vi "Connect.vi"(5 "Connect Meta":T4={"QoS"=enum."At most once", "DUP"=FALSE, "Retain"=TRUE, "Keep Alive (sec)"=60}, 6 "Client ID":string="LabVIEW_MQTT_Client", 7 "Connect Flags":T7, 8 "error in (no error)":errorcluster, 9 "Will Info":T5={"Will Topic"="Will Topic", "Will Message"="Last Will"}, 10 "User Info":T6={"Username"="User", "Password"="password"}, 11 "MQTT Broker":cluster{"address (IP)":string, "port":u16}={"address (IP)"="broker.mqttdashboard.com", "port"=1883}) -> (0 "error out":errorcluster, 2 "Connection Status":T1=enum."Connection refused: not authorized", 3 "connection ID out":refnum<k5>)   [LabVIEW 2025, in "DAQIO MQTT.lvlib"]
doc: "Connects to an MQTT broker server with required settings. \n\n© 2015 - daq.io, LLC - Peter Adelhardt"
uses:
  DAQIO MQTT.lvlib
  Controls/Connect Flags.ctl
  Controls/User Info.ctl
  Controls/Will Info.ctl
  Controls/DUP_Flag.ctl
  Controls/Retain_Flag.ctl
  Controls/Connection_Return_Codes.ctl
  Controls/Conn_FGV_Cmds.ctl
  Controls/Conn_Stat_FGV_Cmds.ctl
  Controls/MessageType.ctl
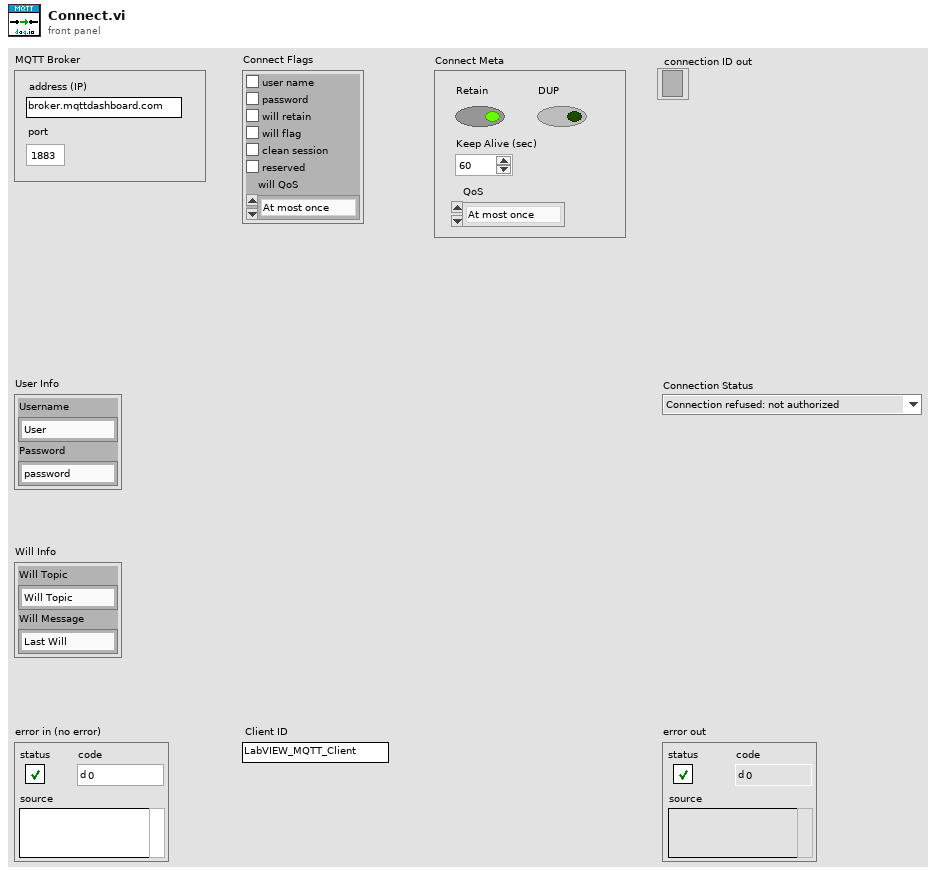
[diagram p1: front panel]
types:
  T1 = typedef "DAQIO MQTT.lvlib/Connection_Return_Codes.ctl" = enum16{"Connection accepted", "Connection refused: unacceptable protocol version", "Connection refused: identifier rejected", "Connection refused: Server unavailable", "Connection refused: bad user name or password", "Connection refused: not authorized"}
  T2 = typedef "DAQIO MQTT.lvlib/DUP_Flag.ctl" = bool
  T3 = typedef "DAQIO MQTT.lvlib/Retain_Flag.ctl" = bool
  T4 = cluster{"QoS":enum8{"At most once", "At least once", "Exactly once", "Reserved"}, "DUP":T2, "Retain":T3, "Keep Alive (sec)":u16}
  T5 = typedef "DAQIO MQTT.lvlib/Will Info.ctl" = cluster{"Will Topic":string, "Will Message":string}
  T6 = typedef "DAQIO MQTT.lvlib/User Info.ctl" = cluster{"Username":string, "Password":string}
  T7 = typedef "DAQIO MQTT.lvlib/Connect Flags.ctl" = cluster{"user name":bool, "password":bool, "will retain":bool, "will flag":bool, "clean session":bool, "reserved":bool, "will QoS":enum8{"At most once", "At least once", "Exactly once", "Reserved"}}
  T8 = typedef "DAQIO MQTT.lvlib/Conn_Stat_FGV_Cmds.ctl" = enum16{"Get", "Set"}
  T9 = typedef "DAQIO MQTT.lvlib/Conn_FGV_Cmds.ctl" = enum16{"Get", "Set", "Delete"}
  T10 = enum8{"At most once", "At least once", "Exactly once", "Reserved"}
  T11 = typedef "DAQIO MQTT.lvlib/MessageType.ctl" = enum32{"Reserved", "CONNECT", "CONNACK", "PUBLISH", "PUBACK", "PUBREC", "PUBREL", "PUBCOMP", "SUBSCRIBE", "SUBACK", "UNSUBSCRIBE", "UNSUBACK", "PINGREQ", "PINGRESP", "DISCONNECT", "Reserved2"}
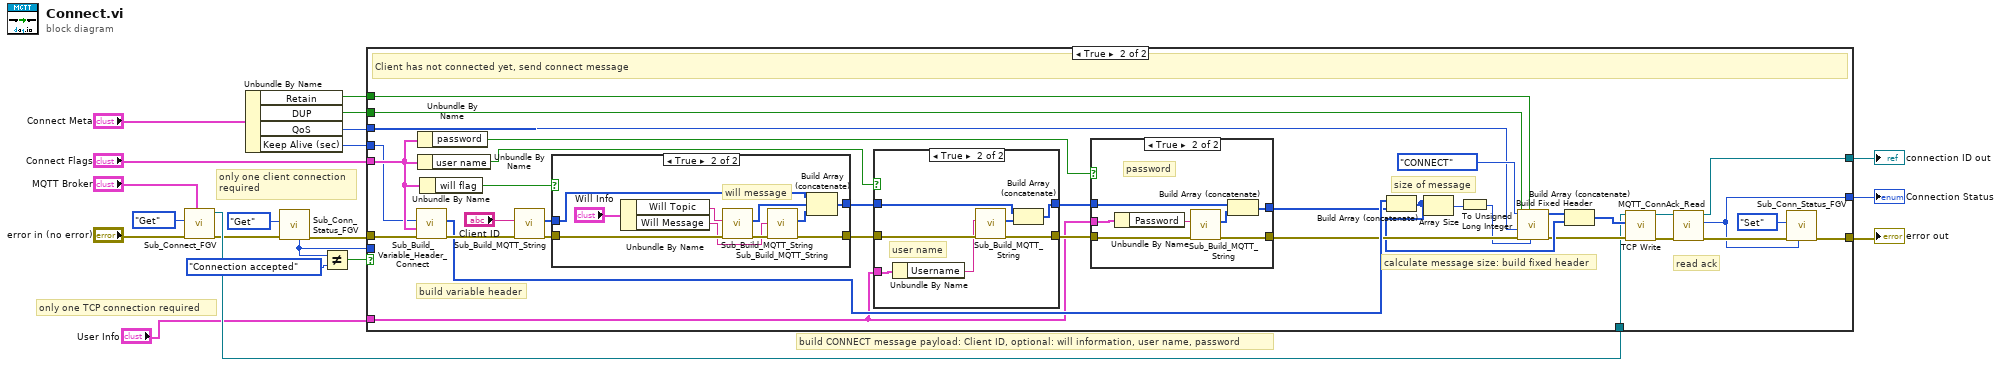
[diagram p0: block diagram]
diagram:
  # "only one client connection\nrequired"
  # "only one TCP connection required"
  # "build CONNECT message payload: Client ID, optional: will information, user name, password"
  n1 = call "Sub_Connect_FGV.vi"("MQTT Broker"="MQTT Broker", "error in"="error in (no error)", "Command"=Conn_FGV_Cmds."Get") -> ("error out"=w6:errorcluster, "Connection ID"=w13:refnum<k5>)  [unwired: 7 in]
  n2 = Unbundle By Name("Connect Meta") -> ("Retain"=w18:T3, "DUP"=w17:T2, "QoS"=w16:T10, "Keep Alive (sec)"=w15:u16)
  n3 = call "Sub_Conn_Status_FGV.vi"("error in"=w6, "Command"=Conn_Stat_FGV_Cmds."Get") -> ("error out"=w3:errorcluster, "Connection Status out"=w2:T1)  [unwired: 8 in]
  n4 = Not Equal?(x=w2, y=Connection_Return_Codes."Connection accepted") -> (x != y?=w4:bool)
  n5 = case shown="True" w4 {
    tunnel: "Connect Flags" -> [_ w53]
    tunnel: w18 -> [_ w40]
    tunnel: w17 -> [_ w39]
    tunnel: w16 -> [_ w38]
    tunnel: w15 -> [_ w37]
    tunnel: w3 -> [w23 w31]
    tunnel: w13 -> [w21 w30]
    tunnel: [w23 w26] -> w10
    tunnel: [w22 w25] -> w9
    tunnel: [w21 w29] -> w8
    tunnel: w2 -> [w22 _]
    tunnel: "User Info" -> [_ w24]
    frame False {
      # "client is already connected"
    }
    frame True {
      # "read ack"
      # "calculate message size: build fixed header"
      # "build variable header"
      # "size of message"
      # "Client has not connected yet, send connect message"
      n6 = call "Sub_Build_Variable_Header_Connect.vi"("error in (no error)"=w31, "Connect Flags"=w53, "Keep Alive (sec)"=w37) -> ("error out"=w58:errorcluster, "Variable Header"=w49:u8[])  [unwired: 7 in]
      n7 = Unbundle By Name(w53) -> ("password"=w51:bool)
      n8 = Unbundle By Name(w53) -> ("user name"=w52:bool)
      n9 = Unbundle By Name(w53) -> ("will flag"=w50:bool)
      n10 = call "Sub_Build_MQTT_String.vi"("error in (no error)"=w58, "String to be encoded"="Client ID") -> ("error out"=w54:errorcluster, "UTF8 Byte Array"=w57:u8[])  [unwired: 8 in]
      n11 = case shown="True" w50 {
        tunnel: w57 -> [w79 w87]
        tunnel: [w79 w88] -> w56
        tunnel: w54 -> [w78 w86]
        tunnel: [w78 w83] -> w47
        frame False {
        }
        frame True {
          # "will message"
          n12 = Unbundle By Name("Will Info") -> ("Will Topic"=w81:string, "Will Message"=w80:string)
          n13 = call "Sub_Build_MQTT_String.vi"("error in (no error)"=w86, "String to be encoded"=w81) -> ("error out"=w85:errorcluster, "UTF8 Byte Array"=w84:u8[])  [unwired: 8 in]
          n14 = call "Sub_Build_MQTT_String.vi"("error in (no error)"=w85, "String to be encoded"=w80) -> ("error out"=w83:errorcluster, "UTF8 Byte Array"=w89:u8[])  [unwired: 8 in]
          n15 = Build Array (concatenate)(w87, w84, w89) -> (w88:u8[])
        }
      }
      n16 = case shown="True" w52 {
        tunnel: w56 -> [w70 w76]
        tunnel: [w70 w75] -> w55
        tunnel: [w69 w74] -> w48
        tunnel: w47 -> [w69 w73]
        tunnel: w24 -> [_ w72]
        frame False {
        }
        frame True {
          # "user name"
          n17 = Unbundle By Name(w72) -> ("Username"=w71:string)
          n18 = call "Sub_Build_MQTT_String.vi"("error in (no error)"=w73, "String to be encoded"=w71) -> ("error out"=w74:errorcluster, "UTF8 Byte Array"=w77:u8[])  [unwired: 8 in]
          n19 = Build Array (concatenate)(w76, w77) -> (w75:u8[])
        }
      }
      n20 = case shown="True" w51 {
        tunnel: w55 -> [w61 w67]
        tunnel: [w61 w66] -> w45
        tunnel: w48 -> [w60 w65]
        tunnel: [w60 w64] -> w46
        tunnel: w24 -> [_ w63]
        frame False {
        }
        frame True {
          # "password"
          n21 = Unbundle By Name(w63) -> ("Password"=w62:string)
          n22 = call "Sub_Build_MQTT_String.vi"("error in (no error)"=w65, "String to be encoded"=w62) -> ("error out"=w64:errorcluster, "UTF8 Byte Array"=w68:u8[])  [unwired: 8 in]
          n23 = Build Array (concatenate)(w67, w68) -> (w66:u8[])
        }
      }
      n24 = Build Array (concatenate)(w49, w45) -> (w44:u8[])
      n25 = Array Size(array=w44) -> (size(s)=w42:i32)
      n26 = To Unsigned Long Integer(number=w42) -> (unsigned 32bit integer=w41:u32)
      n27 = call "Build Fixed Header.vi"("Remaining Length"=w41, "Retain"=w40, "error in (no error)"=w46, "QoS"=w38, "DUP"=w39, "MessageType"=MessageType."CONNECT") -> ("error out"=w35:errorcluster, "Fixed Header"=w43:u8[])  [unwired: 4 in]
      n28 = Build Array (concatenate)(w43, w44) -> (w34:u8[])
      n29 = call "TCP Write.vi"("error in (no error)"=w35, "data in"=w34, "connection ID"=w30) -> ("error out"=w33:errorcluster, "connection ID out"=w32:refnum<k5>)  [unwired: 6 in, 1 out]
      n30 = call "MQTT_ConnAck_Read.vi"("error in (no error)"=w33, "connection ID"=w32) -> ("error out"=w28:errorcluster, "Connection Status"=w25:T1, "connection ID out"=w29:refnum<k5>)  [unwired: 5 in, 2 out]
      n31 = call "Sub_Conn_Status_FGV.vi"("Connection Status in"=w25, "error in"=w28, "Command"=Conn_Stat_FGV_Cmds."Set") -> ("error out"=w26:errorcluster)  [unwired: 7 in, 1 out]
    }
  }
  "error out" <- w10
  "connection ID out" <- w8
  "Connection Status" <- w9
